vi "parse_dataframe.vi"(11 "dataframe":string) -> (3 "DataFrame.lvclass":refnum<class "DataFrame.lvclass">)   [LabVIEW 2017, in "DataFrame.lvclass"]
uses:
  DataFrame.lvclass
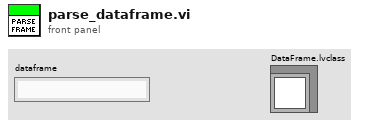
[diagram p1: front panel]
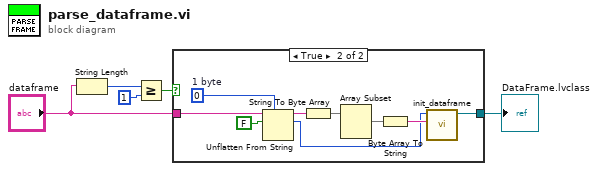
[diagram p0: block diagram]
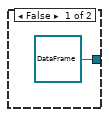
[diagram p2: hidden frame]
diagram:
  n1 = String Length(string="dataframe") -> (length=w4:i32)
  n2 = Greater Or Equal?(x=w4, y=1) -> (x >= y?=w2:bool)
  n3 = case shown="True" w2 {
    tunnel: "dataframe" -> [_ w10]
    tunnel: [refnum<class "DataFrame.lvclass"> refnum ("DataFrame.lvclass") w9] -> w1
    frame False {
    }
    frame True {
      w15 = u8 0  # 1 byte
      n4 = Unflatten From String(type=w15, binary string=w10, data includes array or string size? (T)=FALSE) -> (rest of the binary string=w8:string, value=w7:u8)  [unwired: 2 in, 1 out]
      n5 = String To Byte Array(string=w8) -> (unsigned byte array=w13:u8[])
      n6 = Array Subset(array=w13) -> (w12:u8[])  [unwired: 2 in]
      n7 = Byte Array To String(unsigned byte array=w12) -> (string=w11:string)
      n8 = call "init_dataframe.vi"("data"=w11, "type"=w7) -> ("DataFrame.lvclass"=w9:refnum<class "DataFrame.lvclass">)  [unwired: 9 in]
    }
  }
  "DataFrame.lvclass" <- w1
